vi "Stop FPGA Acquisition.vi"(8 "Error In":errorcluster) -> (0 "Error Out":errorcluster, 3 "FPGA Ref":T1)   [LabVIEW 2013]
doc: "Stops the acquisition."
uses:
  RIG-SPECIFIC FILES/FPGA Refs/FPGA Ref.ctl
  Typedefs/HW config states enum.ctl
  <vilib>/rvi/interface/common/niFpgaWaitOnOcc.vi
  <vilib>/Utility/error.llb/Error Cluster From Error Code.vi
  <vilib>/rvi/interface/nirviMethod/nirviMethod.xnode
  <vilib>/rvi/errors/niLvFpgaMergeErrorWithErrorCode.vi
  <vilib>/FPGAPlugInAG/Dynamic/niLvFpga_StopFifo_Dynamic.vi
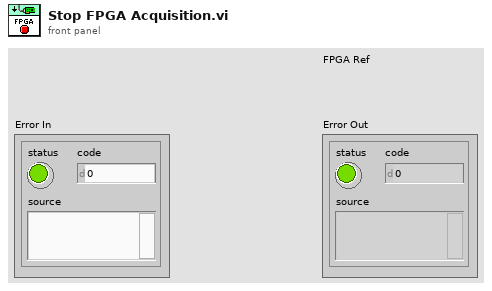
[diagram p1: front panel]
types:
  T1 = typedef "FPGA Ref.ctl" = refnum<k20>
  T2 = typedef "HW config states enum.ctl" = enum16{"Load from file", "Save to file", "Write all", "Read all", "Write XY stage settings", "Write DAQ FPGA settings", "Write Control FPGA settings", "Write Phys Channels", "Clear", "Compare from file"}
  T3 = typedef "Sys Configuration.ctl" = cluster{"XY Stage":T4, "DAQ FPGA":T5, "Control system":T8, "Encoder":T9, "DAQmx Chan":T10, "Computer MAC address":string, "Cam VidRec":T11, "Externalise Triggers":bool, "Laser wavelength (nm)":dbl}
  T4 = typedef "XY Stage config cluster.ctl" = cluster{"COM port":refnum<visa-resource-name>, "XY stage available":bool}
  T5 = typedef "DAQ FPGA config cluster.ctl" = cluster{"Ref":T1, "Target":T6, "Clock Freq (MHz) ":dbl, "input card type":T7, "Samples Wait after Trigger":u16, "AOD fill":u16, "StartupDelay":i32, "Slip Cycle (clock cycles)":u32, "Add Cycle":bool}
  T6 = typedef "nirio_resource_hc.ctl" = tag
  T7 = typedef "FPGA input type AC-DC.ctl" = enum16{"AC Card", "DC Card"}
  T8 = typedef "CTRL system config cluster.ctl" = cluster{"Ethernet opened":bool, "Ethernet Port":u32, "Ctrl FPGA available":bool, "Ctrl FPGA Clock (MHz)":dbl, "Ctrl system MAC address":string, "Control system.Network adapter name":string, "AOD 1 Amplitude":i16, "AOD 2 Amplitude":i16, "AOD 3 Amplitude":i16, "AOD 4 Amplitude":i16, "Data Time Interval (ns)":dbl, "T0 (ns)":dbl, "Ta (ns)":dbl}
  T9 = typedef "Encoder config cluster.ctl" = cluster{"IP address":string, "Port":u16, "Encoder available":bool, "Wheel radius (cm)":dbl}
  T10 = typedef "DAQmx physical channels cluster.ctl" = cluster{"Pockels AO":tag, "Hard shutter AO":tag, "PMT AOs":tag, "Power meter AI":tag}
  T11 = typedef "Cam VidRec HW config setup cluster.ctl" = cluster{"DO flag-Video record":tag, "DO flag-Trial start":tag, "VidRec available":bool}
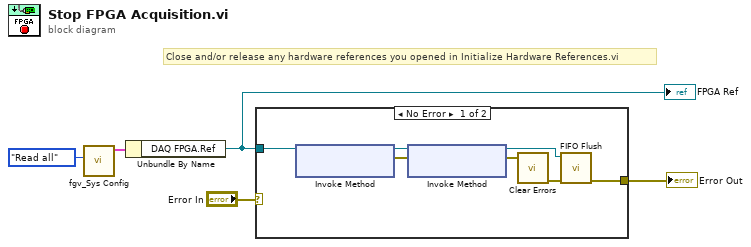
[diagram p0: block diagram]
diagram:
  # "Close and/or release any hardware references you opened in Initialize Hardware References.vi"
  n1 = call "fgv_Sys Config.vi"("Function"=HW_config_states_enum."Read all") -> ("System Config out"=w3:T3)  [unwired: 9 in, 1 out]
  n2 = Unbundle By Name(w3) -> ("DAQ FPGA.Ref"=w1:T1)
  "FPGA Ref" <- w1
  n3 = case shown="No Error" "Error In" {
    selector: "Error In" -> [_ w13]
    tunnel: [w6 w13] -> w4
    tunnel: w1 -> [w7 _]
    frame No Error {
      n4 = xnode "Invoke Method"("FPGA VI Reference In"=w7) -> ("FPGA VI Reference Out"=w11:T1, "error out"=w10:errorcluster)  [unwired: 1 in]
      n5 = xnode "Invoke Method"("FPGA VI Reference In"=w11, "error in"=w10) -> ("FPGA VI Reference Out"=w8:T1, "error out"=w12:errorcluster)
      n6 = call <vilib>:"Clear Errors.vi"("error in (no error)"=w12) -> ("error out"=w9:errorcluster)  [unwired: 6 in]
      n7 = call "FIFO Flush.vi"("Error In"=w9, "FPGA VI Ref"=w8) -> ("Error Out"=w6:errorcluster)  [unwired: 7 in, 2 out]
    }
    frame Error {
    }
  }
  "Error Out" <- w4
